vi "Set Aircraft COM Port.vi"(7 "Downlink(T)/Uplink(f)":bool, 8 "Error In":errorcluster, 10 "COM Port":refnum<visa-resource-name>, 11 "Aircraft ID":u8) -> (0 "Error Out":errorcluster)   [LabVIEW 2014]
uses:
  Get Aircraft Information.vi
  Set Aircraft Information.vi
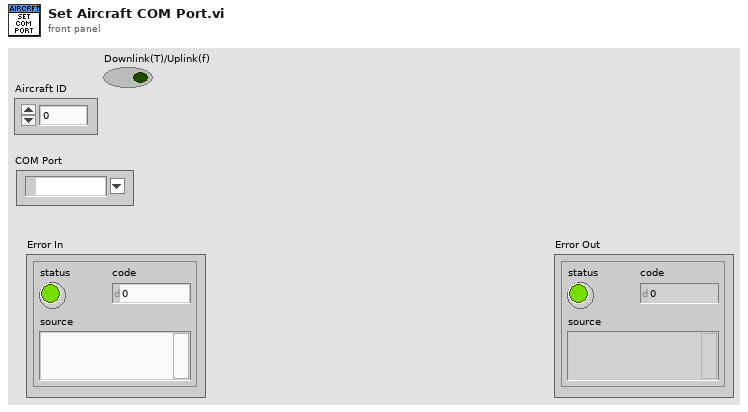
[diagram p1: front panel]
types:
  T1 = typedef "Drone Information.ctl" = cluster{"Heart Beat":bool, "Aircraft ID":u8, "Downlink Port":refnum<visa-resource-name>, "Tag ID":string, "System Status":string, "Base Mode":T2, "Armed/Disarmed":bool, "Battery Voltage":dbl, "Control Mode":T3, "Initialisation":u8, "Heart Beat Status":bool, "Uplink Port":refnum<visa-resource-name>, "UDP connection ID":refnum<k16>, "Connection Type":T4, "Mode":string, "UDP IP Address":string, "Mission Uploaded":bool}
  T2 = typedef "Base Mode.ctl" = cluster{"Custom Mode":bool, "Test Enabled":bool, "Autonomous Mode":bool, "Guided Mode":bool, "Stabilization Enabled":bool, "HIL Enabled":bool, "Manual Mode":bool, "Arm":bool}
  T3 = typedef "Aircraft Mode.ctl" = enum16{"Loiter", "Stabalise", "Failsafe", "Emergency Stop"}
  T4 = typedef "Telemetry Connection Type.ctl" = enum16{"Serial", "UDP", "TCP"}
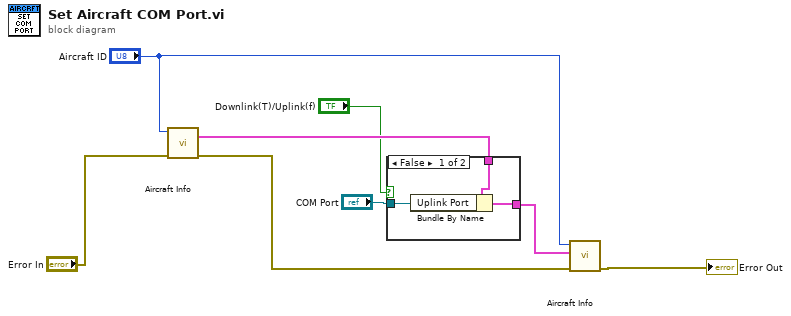
[diagram p0: block diagram]
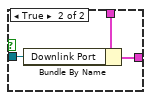
[diagram p2: hidden frame]
diagram:
  n1 = call-poly "Aircraft Info.vi"("Error In"="Error In", "Aircraft ID"="Aircraft ID") -> ("Error Out"=w6:errorcluster, "Aircraft Information Out"=w8:T1)  [unwired: 8 in]
  n2 = case shown="False" "Downlink(T)/Uplink(f)" {
    tunnel: w8 -> [w10 w14]
    tunnel: [w11 w13] -> w7
    tunnel: "COM Port" -> [w9 w12]
    frame False {
      n3 = Bundle By Name(cluster=w10, "Uplink Port"=w9) -> (w11:T1)
    }
    frame True {
      n4 = Bundle By Name(cluster=w14, "Downlink Port"=w12) -> (w13:T1)
    }
  }
  n5 = call-poly "Aircraft Info.vi"("Error In"=w6, "Aircraft Information In"=w7, "Aircraft ID"="Aircraft ID") -> ("Error Out"=→"Error Out":errorcluster)  [unwired: 8 in]
